vi "Tosca-TCP test.vi"() -> ()   [LabVIEW 2020]
panel:
  out "date/time string":string
  out "error out":errorcluster
  in  "command string":string="Time"
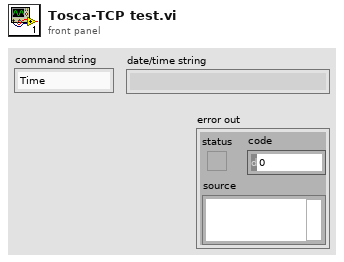
[diagram p1: front panel]
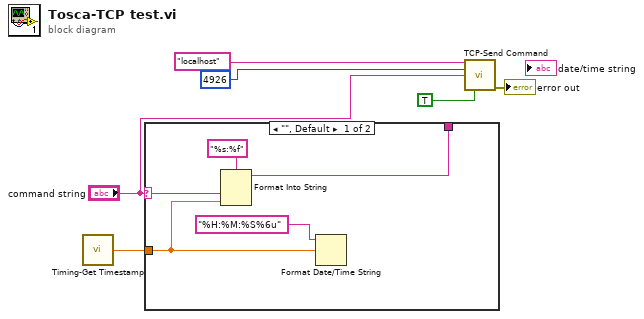
[diagram p0: block diagram]
diagram:
  n1 = call "Timing-Get Timestamp.vi"() -> ("double precision float"=w3:dbl)  [unwired: 14 in, 1 out]
  n2 = case shown="\"\", Default" "command string" {
    selector: "command string" -> [w10 w12]
    tunnel: [w9 w12] -> _
    tunnel: w3 -> [w7 _]
    frame "", Default {
      n3 = Format Into String(format string="%s:%f", w10, w7) -> (resulting string=w9:string)  [unwired: 2 in, 1 out]
      n4 = Format Date/Time String(time format string (%c)="%H:%M:%S%6u", seconds (now)=w7) -> ()  [unwired: 1 in, 1 out]
    }
    frame "Quit" {
    }
  }
  n5 = call "TCP-Send Command.vi"("PXI Address"="localhost" ("address"), "Port"=u16 4926 ("remote port or service name"), "Command"="command string", "fast response"=TRUE) -> ("error out"=→"error out":errorcluster)  [unwired: 11 in]
